vi "TCP-Enable-broadcasting.vi"() -> ()   [LabVIEW 2013, in "HardwareCharacterization.lvlib" / "HC-SM1000.lvclass"]
uses:
  HC-SM1000.lvclass
  Hosts.ctl
  TCP-settings.ctl
  Broadcasting.ctl
panel:
  in  "Broadcasting":T1=enum."Enable"
  out "TCP settings":T2={"Target IP"="128.178.146.163", "Target TCP port"=12500, "TCP read mode"=enum."CRLF", "TCP read buffer"=4096, "Read timeout"=5000}
  out "Host in control":T3=enum."Pendant"
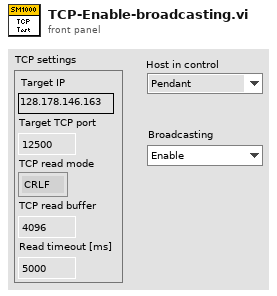
[diagram p1: front panel]
types:
  T1 = typedef "HardwareCharacterization.lvlib/HC-SM1000.lvclass/Broadcasting.ctl" = enum16{"Disable", "Enable"}
  T2 = typedef "HardwareCharacterization.lvlib/HC-SM1000.lvclass/TCP-settings.ctl" = cluster{"Target IP":string, "Target TCP port":u16, "TCP read mode":enum16{"Standard", "Buffered", "CRLF", "Immediate"}, "TCP read buffer":i32, "Read timeout":i32}
  T3 = typedef "HardwareCharacterization.lvlib/HC-SM1000.lvclass/Hosts.ctl" = enum16{"None", "Pendant", "LANStream", "LAN"}
  T4 = typedef "HardwareCharacterization.lvlib/HC-SM1000.lvclass/Object-reference.ctl" = refnum<data-value>
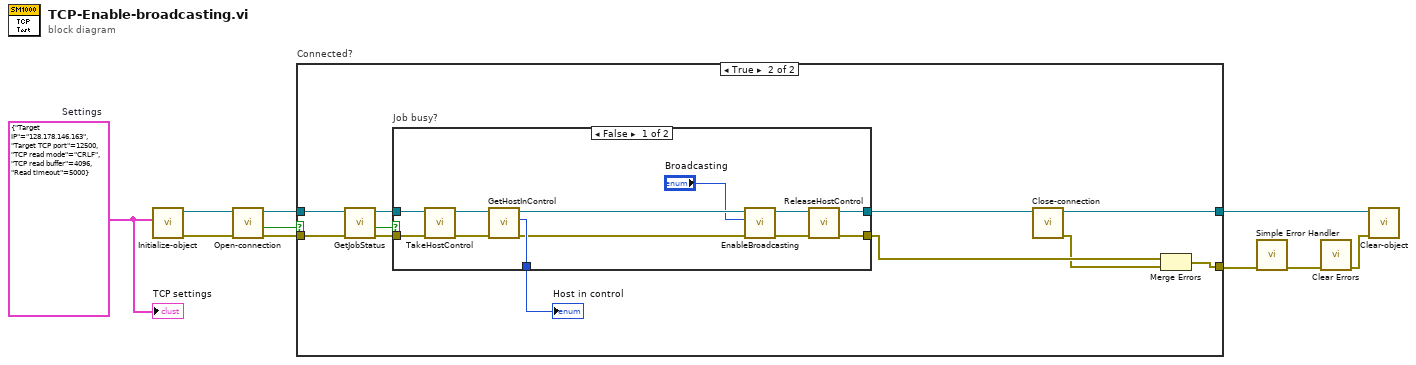
[diagram p0: block diagram]
diagram:
  w10 = T2 {"Target IP"="128.178.146.163", "Target TCP port"=12500, "TCP read mode"=enum."CRLF", "TCP read buffer"=4096, "Read timeout"=5000}  # Settings
  n1 = call "Initialize-object.vi"("TCP settings"=w10) -> ("error out"=w8:errorcluster, "SM1000-control out"=w9:T4)  [unwired: 9 in]
  n2 = call "Open-connection.vi"("error in (no error)"=w8, "SM1000-control in"=w9) -> ("error out"=w6:errorcluster, "Connected?"=w5:bool, "SM1000-control out"=w7:T4)  [unwired: 7 in]
  n3 = case "Connected?" shown="True" w5 {
    tunnel: w7 -> [w11 w14]
    tunnel: w6 -> [w12 w13]
    tunnel: [w12 w16] -> w3
    tunnel: [w11 w15] -> w2
    frame False {
    }
    frame True {
      n4 = call "GetJobStatus.vi"("error in (no error)"=w13, "SM1000-control in"=w14) -> ("error out"=w21:errorcluster, "Busy?"=w23:bool, "SM1000-control out"=w22:T4)  [unwired: 7 in]
      n5 = case "Job busy?" shown="False" w23 {
        tunnel: w22 -> [w35 w37]
        tunnel: w21 -> [w34 w36]
        tunnel: [w31 _] -> w20
        tunnel: [w30 w37] -> w19
        tunnel: [w29 w36] -> w18
        frame False {
          n6 = call "TakeHostControl.vi"("error in (no error)"=w34, "SM1000-control in"=w35) -> ("error out"=w32:errorcluster, "SM1000-control out"=w33:T4)  [unwired: 8 in]
          n7 = call "GetHostInControl.vi"("error in (no error)"=w32, "SM1000-control in"=w33) -> ("error out"=w25:errorcluster, "Host in control"=w31:T3, "SM1000-control out"=w28:T4)  [unwired: 7 in]
          n8 = call "EnableBroadcasting.vi"("error in (no error)"=w25, "Broadcasting"="Broadcasting", "SM1000-control in"=w28) -> ("error out"=w26:errorcluster, "SM1000-control out"=w27:T4)  [unwired: 7 in]
          n9 = call "ReleaseHostControl.vi"("error in (no error)"=w26, "SM1000-control in"=w27) -> ("error out"=w29:errorcluster, "SM1000-control out"=w30:T4)  [unwired: 8 in]
        }
        frame True {
        }
      }
      "Host in control" <- w20
      n10 = call "Close-connection.vi"("SM1000-control in"=w19) -> ("error out"=w17:errorcluster, "SM1000-control out"=w15:T4)  [unwired: 8 in, 1 out]
      n11 = Merge Errors(w18, w17) -> (w16:errorcluster)
    }
  }
  n12 = call <vilib>:"Simple Error Handler.vi"("error in (no error)"=w3) -> ("error out"=w4:errorcluster)  [unwired: 4 in, 4 out]
  n13 = call <vilib>:"Clear Errors.vi"("error in (no error)"=w4) -> ("error out"=w1:errorcluster)  [unwired: 6 in]
  n14 = call "Clear-object.vi"("error in (no error)"=w1, "SM1000-control"=w2) -> ()  [unwired: 8 in, 2 out]
  "TCP settings" <- w10
